vi "F Dwf Analog Out Trigger Slope Set.vi"(8 "error in (no error)":errorcluster, 9 "slope":i32, 10 "idxChannel":i32, 11 "hdwf":i32) -> (0 "error out":errorcluster, 3 "function return":i32)   [LabVIEW 2019, in "Olasdwf.lvlib"]
doc: "DWFAPI int FDwfAnalogOutTriggerSlopeSet(HDWF hdwf, int idxChannel, DwfTriggerSlope slope);"
uses:
  Olasdwf.lvlib
  Windows/System32/dwf.dll
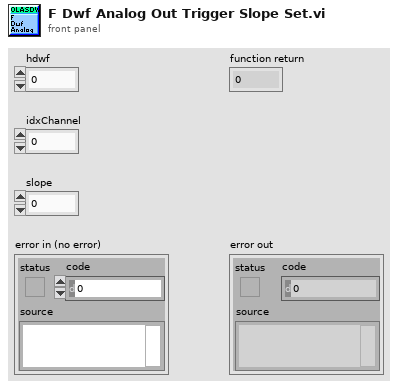
[diagram p1: front panel]
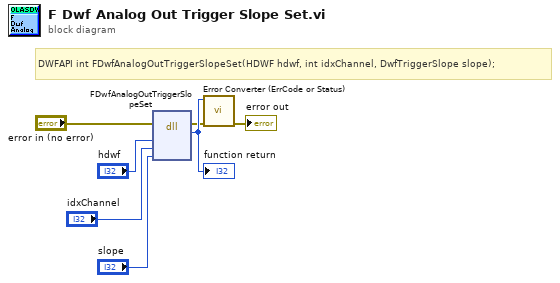
[diagram p0: block diagram]
diagram:
  # "DWFAPI int FDwfAnalogOutTriggerSlopeSet(HDWF hdwf, int idxChannel, DwfTriggerSlope slope);"
  n1 = dll-call lib="C:/Windows/System32/dwf.*" fn="FDwfAnalogOutTriggerSlopeSet"(error in="error in (no error)", "hdwf"="hdwf", "idxChannel"="idxChannel", "slope"="slope") -> (error out=w2:errorcluster, w7:i32)  [unwired: 5 in, 1 out]
  "function return" <- w7
  n2 = call "Error Converter (ErrCode or Status).vi"("error in (no error)"=w2, "error code"=w7) -> ("error out"=→"error out":errorcluster)  [unwired: 9 in]
